vi "ChartsAndGraphs-unfinished.vi"() -> ()   [LabVIEW 2014]
panel:
  in  "stop":bool
  in  "time step (s)":dbl=0.25
  in  "phase":dbl format="%0.2f"
  in  "frequency":dbl=0.5 format="%0.2f"
  in  "amplitude":dbl=1.0 format="%0.2f"
  # "Sine wave"
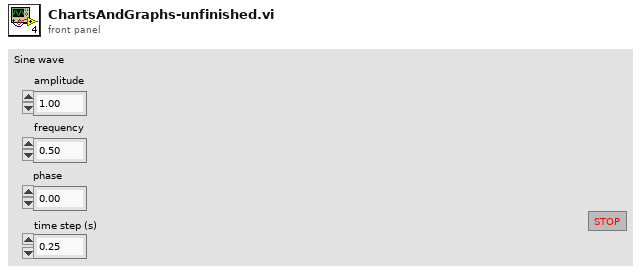
[diagram p1: front panel]
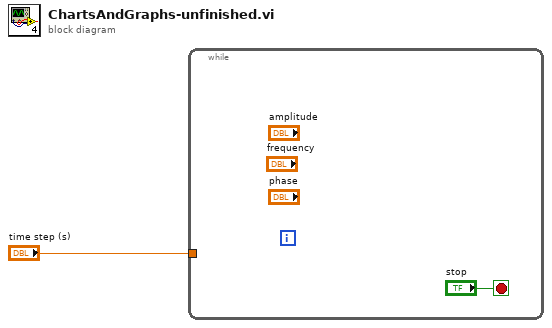
[diagram p0: block diagram]
diagram:
  n1 = while {
    tunnel: "time step (s)" -> [_]
    stop <- "stop" stop-if-true
  }
